vi "RSZVB Set External Signal Source AUX.vi"(8 "error in (no error)":errorcluster {"code" format="%.0x"}, 9 "External Signal Source (0)":i32, 10 "Channel (1)":i32=1, 11 "VISA session":refnum<visa-resource-name>) -> (0 "error out":errorcluster {"code" format="%.0x"}, 3 "dup VISA session":refnum<visa-resource-name>)   [LabVIEW 2011]
doc: "Selects an external generator as a signal source for the Aux LO signal in a vector mixer measurement (option R&S ZVA-K5). The Aux LO signal is fed to the MEAS and REF mixers.\n\nRemote-control command(s):\n[SENSe<Ch>:]FREQuency:CONVersion:MIXer:AEXTernal NONE | <port_number>"
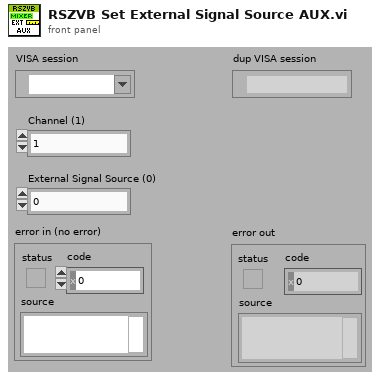
[diagram p1: front panel]
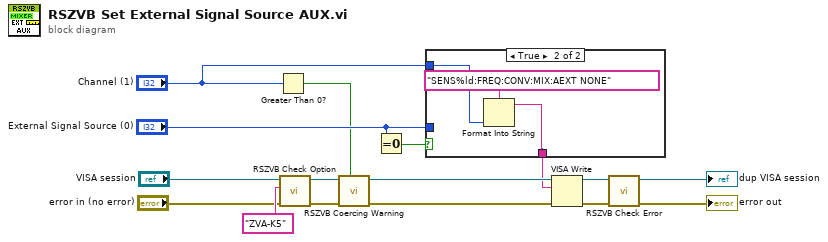
[diagram p0: block diagram]
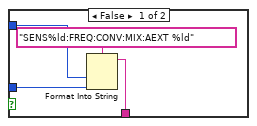
[diagram p2: hidden frame]
diagram:
  n1 = Greater Than 0?(x="Channel (1)") -> (x > 0?=w1:bool)
  n2 = call "RSZVB Check Option.vi"("error in (no error)"="error in (no error)", "Options"="ZVA-K5", "VISA session"="VISA session") -> ("error out"=w8:errorcluster, "dup VISA session"=w9:refnum<visa-resource-name>)  [unwired: 7 in]
  n3 = call "RSZVB Coercing Warning.vi"("In Range?"=w1, "error in (no error)"=w8, "VISA session"=w9) -> ("error out"=w15:errorcluster, "dup VISA session"=w16:refnum<visa-resource-name>)  [unwired: 7 in]
  n4 = Equal To 0?(x="External Signal Source (0)") -> (x = 0?=w11:bool)
  n5 = case shown="True" w11 {
    tunnel: [w19 w22] -> w12
    tunnel: "External Signal Source (0)" -> [w18 _]
    tunnel: "Channel (1)" -> [w17 w21]
    frame False {
      n6 = Format Into String(format string="SENS%ld:FREQ:CONV:MIX:AEXT %ld", w17, w18) -> (resulting string=w19:string)  [unwired: 2 in, 1 out]
    }
    frame True {
      n7 = Format Into String(format string="SENS%ld:FREQ:CONV:MIX:AEXT NONE", w21) -> (resulting string=w22:string)  [unwired: 2 in, 1 out]
    }
  }
  n8 = VISA Write(VISA resource name=w16, write buffer=w12, error in (no error)=w15) -> (VISA resource name out=w13:refnum<visa-resource-name>, error out=w14:errorcluster)  [unwired: 1 out]
  n9 = call "RSZVB Check Error.vi"("error in (no error)"=w14, "VISA session"=w13) -> ("error out"=→"error out":errorcluster, "dup VISA session"=→"dup VISA session":refnum<visa-resource-name>)  [unwired: 8 in]
